vi "Event_timestamp.vi"() -> (3 "date/time string":string, 7 "Raw time output":dbl)   [LabVIEW 2017, in "labview-standard-library.lvlib" / "data-logging.lvlib"]
uses:
  data-logging.lvlib
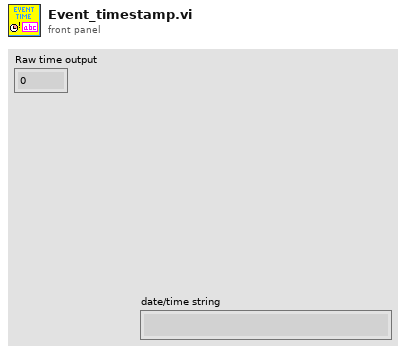
[diagram p1: front panel]
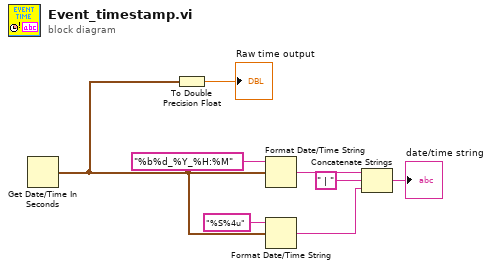
[diagram p0: block diagram]
diagram:
  n1 = Get Date/Time In Seconds() -> (seconds since 1Jan1904=w2:timestamp)
  n2 = To Double Precision Float(number=w2) -> (double precision float=→"Raw time output":dbl)
  n3 = Format Date/Time String(time format string (%c)="%b%d_%Y_%H:%M" ("Event log time format string"), seconds (now)=w2) -> (date/time string=w6:string)  [unwired: 1 in]
  n4 = Format Date/Time String(time format string (%c)="%S%4u", seconds (now)=w2) -> (date/time string=w5:string)  [unwired: 1 in]
  n5 = Concatenate Strings(w6, " | " ("string"), w5) -> (→"date/time string":string)
